vi "Close Error Task_Manager.vi"(8 "error in (no error)":errorcluster, 11 "Error Task Manager in":refnum<class "Error Task Manager.lvclass">) -> (0 "error out":errorcluster)   [LabVIEW 2013, in "Error Task Manager.lvlib" / "Error Task Manager.lvclass"]
doc: "This vi Close Task Manager Error"
uses:
  Error Task Manager.lvclass
  Error Task Manager.lvclass/Error Task Manager.ctl
panel:
  out "Error Task Manager out":refnum<class "Error Task Manager.lvclass">
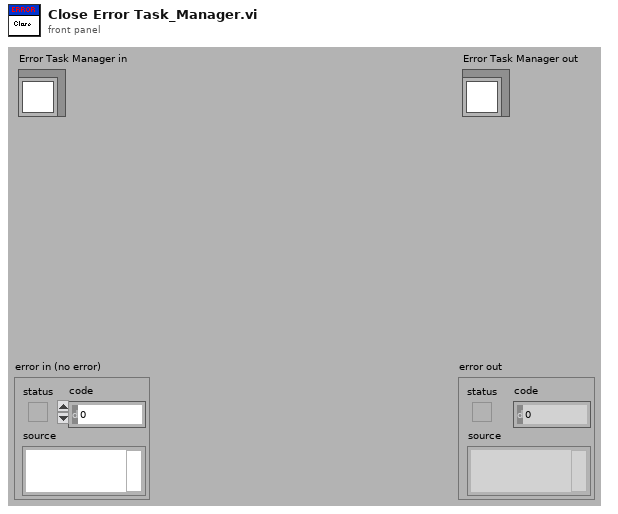
[diagram p1: front panel]
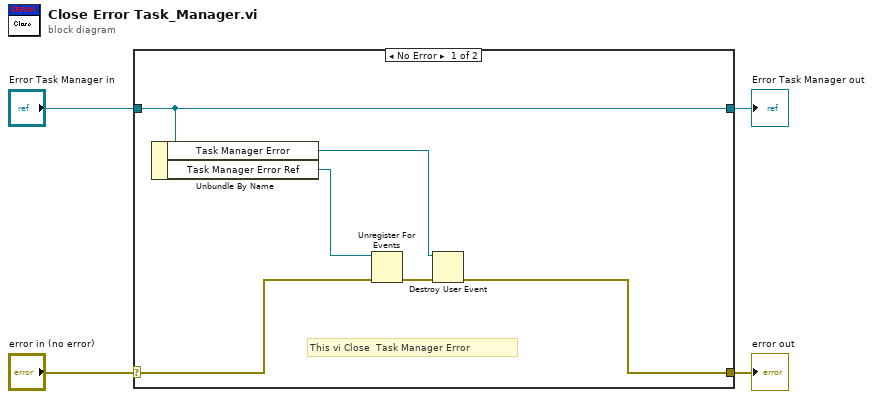
[diagram p0: block diagram]
diagram:
  n1 = case shown="No Error" "error in (no error)" {
    selector: "error in (no error)" -> [w6 w12]
    tunnel: [w5 w12] -> w3
    tunnel: [w10 w11] -> w1
    tunnel: "Error Task Manager in" -> [w10 w11]
    frame No Error {
      # "This vi Close  Task Manager Error"
      n2 = Unbundle By Name(w10) -> ("Task Manager Error"=w7:refnum<user-event>, "Task Manager Error Ref"=w9:refnum<event-registration>)
      n3 = Unregister For Events(event registration refnum=w9, error in=w6) -> (error out=w8:errorcluster)
      n4 = Destroy User Event(user event=w7, error in=w8) -> (error out=w5:errorcluster)
    }
    frame Error {
    }
  }
  "error out" <- w3
  "Error Task Manager out" <- w1
